vi "ke37xx Get Channel Status.vi"(0 "VISA Resource Name":refnum<visa-resource-name>, 1 "Channel":string, 11 "error in (no error)":errorcluster, 12 "Bytes To Read (1024)":u32=1024) -> (4 "VISA Resource Name Out":refnum<visa-resource-name>, 6 "Closure Count":i32, 8 "Associated Channels":string, 15 "error out":errorcluster)   [LabVIEW 2009, in "Keithley 3700 Series.lvlib"]
doc: "This VI queies a channel for its closure count and for its associated channels and analog backplane relays."
uses:
  <instrlib>/Keithley 3706/Keithley 3700 Series.lvlib
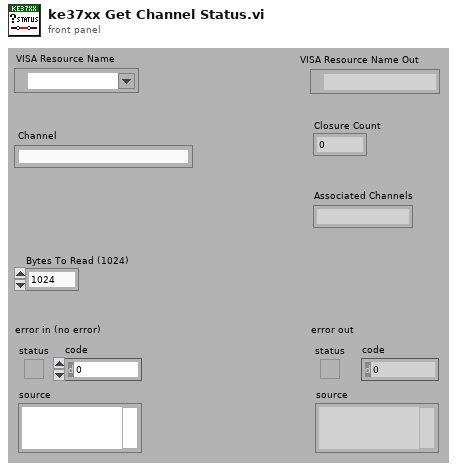
[diagram p1: front panel]
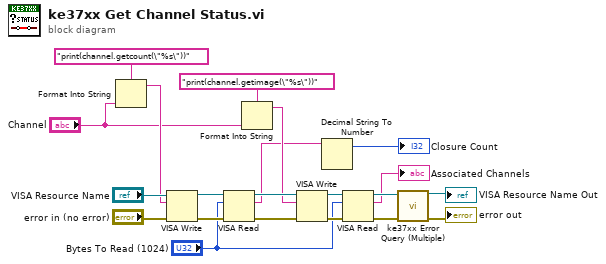
[diagram p0: block diagram]
diagram:
  n1 = Format Into String(format string="print(channel.getcount(\"%s\"))", "Channel") -> (resulting string=w14:string)  [unwired: 2 in, 1 out]
  n2 = VISA Write(VISA resource name="VISA Resource Name", write buffer=w14, error in (no error)="error in (no error)") -> (VISA resource name out=w17:refnum<visa-resource-name>, error out=w16:errorcluster)  [unwired: 1 out]
  n3 = VISA Read(VISA resource name=w17, byte count="Bytes To Read (1024)", error in (no error)=w16) -> (VISA resource name out=w11:refnum<visa-resource-name>, read buffer=w2:string, error out=w10:errorcluster)  [unwired: 1 out]
  n4 = Format Into String(format string="print(channel.getimage(\"%s\"))", "Channel") -> (resulting string=w7:string)  [unwired: 2 in, 1 out]
  n5 = VISA Write(VISA resource name=w11, write buffer=w7, error in (no error)=w10) -> (VISA resource name out=w9:refnum<visa-resource-name>, error out=w8:errorcluster)  [unwired: 1 out]
  n6 = Decimal String To Number(string=w2) -> (offset past number=→"Closure Count":i32)  [unwired: 3 out]
  n7 = VISA Read(VISA resource name=w9, byte count="Bytes To Read (1024)", error in (no error)=w8) -> (VISA resource name out=w6:refnum<visa-resource-name>, read buffer=→"Associated Channels":string, error out=w5:errorcluster)  [unwired: 1 out]
  n8 = call <instrlib>:"ke37xx Error Query (Multiple).vi"("VISA resource name"=w6, "error in (no error)"=w5) -> ("VISA resource name out"=→"VISA Resource Name Out":refnum<visa-resource-name>, "error out"=→"error out":errorcluster)  [unwired: 12 out]
